vi "Read Data from Instrument.vi"(8 "error in (no error)":errorcluster, 10 "Address":string, 11 "heater_parent in":refnum<class "heater_parent.lvclass">) -> (0 "error out":errorcluster, 2 "Value Read":dbl, 3 "heater_parent out":refnum<class "heater_parent.lvclass">)   [LabVIEW 2020, in "polar_bear_plus_drivers.lvlib" / "heater_parent.lvclass"]
doc: "Reads a value from the given address for the instrument."
uses:
  <instrlib>/RxnRover/Driver Polar Bear Plus/heater_parent/heater_parent.lvclass
  <instrlib>/RxnRover/Driver Polar Bear Plus/heater_parent/heater_parent.lvclass/heater_parent.ctl
  <instrlib>/Eurotherm nanodac/Eurotherm nanodac.lvlib
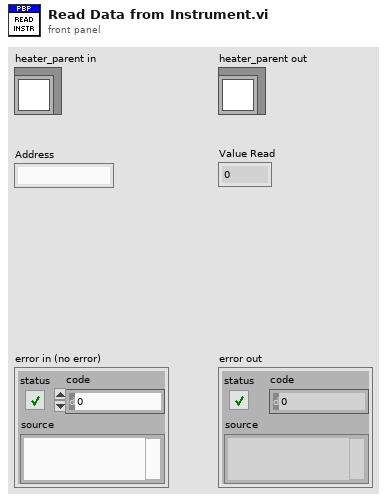
[diagram p1: front panel]
types:
  T1 = typedef "Eurotherm nanodac.lvlib/Parameter Info.ctl" = cluster{"Reference Name":string, "Modbus Address":u16, "Bisynch Mnemonic":string, "Data Type":enum16{"BOOL", "STATE_T", "UINT8", "INT16", "UINT16", "INT32", "UINT32", "TIME_T", "MODBUS_ADDRESS", "FLOAT32", "32BYTES", "EFLOAT32", "ETIME_T", "EINT32", "STRING_T"}, "Availability":string, "Alterability":string, "Low Limit":string, "High Limit":string, "Storage Type":enum16{"RAM", "NON-VOL"}, "Display Resolution":enum16{"0", "1", "2", "PV", "N/A"}, "User Access Conf":enum16{"ALTR", "READ", "HIDE", "N/A"}, "Factory Comms Address":u16, "Enumeration List":string, "Bit Mask":u16, "Description":string}
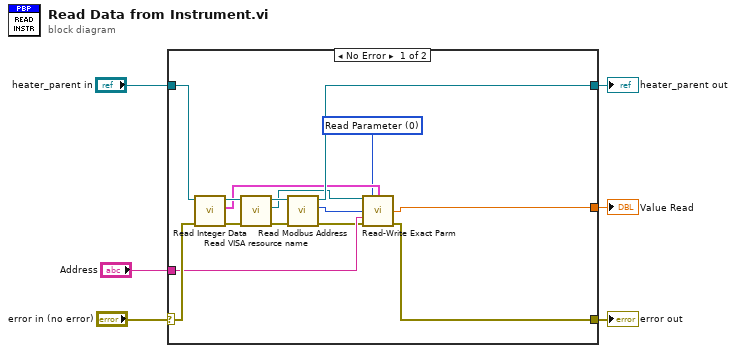
[diagram p0: block diagram]
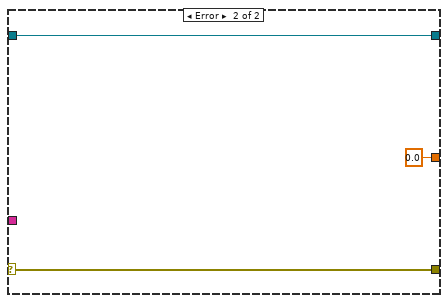
[diagram p2: hidden frame]
diagram:
  n1 = case shown="No Error" "error in (no error)" {
    selector: "error in (no error)" -> [w21 w23]
    tunnel: [w19 0.0 ("Value Read")] -> w1
    tunnel: [w11 w24] -> w6
    tunnel: [w20 w23] -> w5
    tunnel: "Address" -> [w18 _]
    tunnel: "heater_parent in" -> [w14 w24]
    frame No Error {
      w7 = u16 0 items=["Read Parameter", "Write Parameter"] ("Read/Write (0: Read)")
      n2 = call-dynamic "Read Integer Data.vi"("error in (no error)"=w21, "heater_parent in"=w14) -> ("error out"=w17:errorcluster, "Integer Data"=w8:T1[], "heater_parent out"=w13:refnum<class "heater_parent.lvclass">)  [unwired: 7 in]
      n3 = call-dynamic "Read VISA resource name.vi"("error in (no error)"=w17, "vici_flow_actuator_parent in"=w13) -> ("error out"=w16:errorcluster, "VISA resource name"=w9:refnum<visa-resource-name>, "vici_flow_actuator_parent out"=w12:refnum<class "heater_parent.lvclass">)  [unwired: 7 in]
      n4 = call-dynamic "Read Modbus Address.vi"("error in (no error)"=w16, "heater_parent in"=w12) -> ("error out"=w15:errorcluster, "Modbus Address"=w10:u8, "heater_parent out"=w11:refnum<class "heater_parent.lvclass">)  [unwired: 7 in]
      n5 = call <instrlib>:"Read-Write Exact Parm.vi"("VISA resource name"=w9, "Read/Write (0: Read)"=w7, "Integer Data"=w8, "Unit Address (1)"=w10, "Reference Name"=w18, "error in (no error)"=w15) -> ("Value Read"=w19:dbl, "error out"=w20:errorcluster)  [unwired: 4 in, 4 out]
    }
    frame Error {
    }
  }
  "heater_parent out" <- w6
  "error out" <- w5
  "Value Read" <- w1
